vi "RemoveZeros.vi"() -> ()   [LabVIEW 2011]
panel:
  out "Size":i32
  out "ExecTime":u32
  in  "Valeur à enlever":dbl=255.0
  out "Nb trouvées":i32
  out "Output Array":dbl[](array[numeric])
  in  "Input aArray":dbl[](array[numeric])
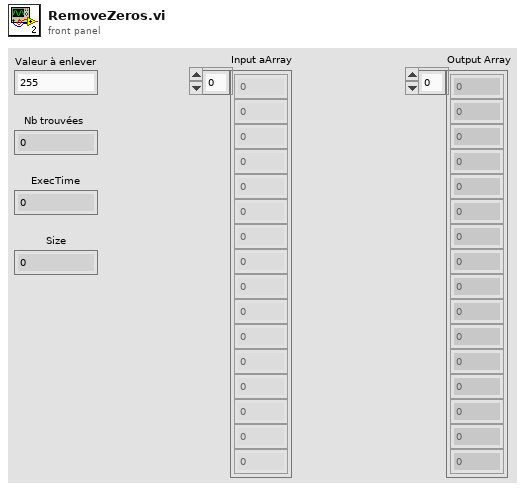
[diagram p1: front panel]
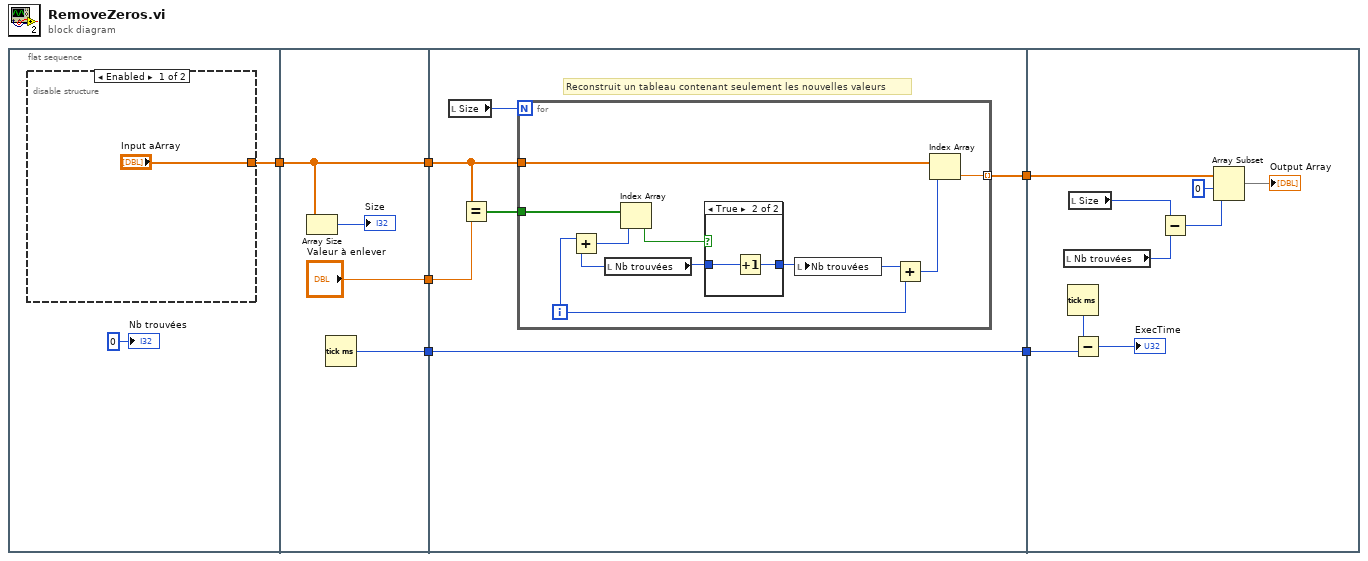
[diagram p0: block diagram]
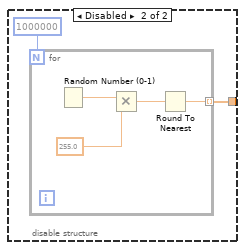
[diagram p2: hidden frame]
diagram:
  n1 = flat-sequence {
    tunnel: [w8] -> w6
    tunnel: w6 -> [w17]
    tunnel: [w17] -> w5
    tunnel: ["Valeur à enlever"] -> w4
    tunnel: [w18] -> w2
    tunnel: w5 -> [w24]
    tunnel: w4 -> [w23]
    tunnel: [w22] -> w3
    tunnel: w2 -> [w22]
    tunnel: [w20] -> w1
    tunnel: w3 -> [w46]
    tunnel: w1 -> [w40]
    frame #0 {
      n2 = disable-structure shown="Enabled" {
        disable-tunnel: ["Input aArray" w11] -> w8
        frame Enabled {
        }
        frame Disabled {
          n3 = for {
            N: 1000000 -> [_]
            tunnel: [w12] -> w11 mode=indexing
            n4 = Random Number (0-1)() -> (number: 0 to 1=w15:dbl)
            n5 = Multiply(x=w15, y=255.0) -> (x*y=w13:dbl)
            n6 = Round To Nearest(number=w13) -> (nearest integer value=w12:dbl)
          }
        }
      }
      "Nb trouvées" <- 0 ("Nb Zeros")
    }
    frame #1 {
      n7 = Array Size(array=w17) -> (size(s)=→"Size":i32)
      n8 = Tick Count (ms)() -> (millisecond timer value=w18:u32)
    }
    frame #2 {
      # "Reconstruit un tableau contenant seulement les nouvelles valeurs"
      n9 = local read "Size"() -> (w21:i32)
      n10 = Equal?(x=w24, y=w23) -> (x = y?=w25:bool[])
      n11 = for {
        N: w21 -> [_]
        tunnel: w24 -> [w34]
        tunnel: w25 -> [w29]
        tunnel: [w33] -> w20 mode=indexing
        i -> [w31]
        n12 = local read "Nb trouvées"() -> (w30:i32)
        n13 = Add(x=w31, y=w30) -> (x+y=w27:i32)
        n14 = Index Array(array=w29, index=w27) -> (element=w26:bool)
        n15 = case shown="True" w26 {
          tunnel: w30 -> [w35 w37]
          tunnel: [w35 w36] -> w28
          frame False {
          }
          frame True {
            n16 = Increment(x=w37) -> (x+1=w36:i32)
          }
        }
        n17 = local write "Nb trouvées"(w28) -> ()
        n18 = Add(x=w28, y=w31) -> (x+y=w32:i32)
        n19 = Index Array(array=w34, index=w32) -> (element=w33:dbl)
      }
    }
    frame #3 {
      n20 = local read "Nb trouvées"() -> (w38:i32)
      n21 = Tick Count (ms)() -> (millisecond timer value=w45:u32)
      n22 = local read "Size"() -> (w43:i32)
      n23 = Subtract(x=w45, y=w46) -> (x-y=→"ExecTime":u32)
      n24 = Subtract(x=w43, y=w38) -> (x-y=w42:i32)
      n25 = Array Subset(array=w40, index=0, length=w42) -> (→"Output Array":dbl[])
    }
  }
